vi "Start Action Core.vi"(8 "error in (no error)":errorcluster, 11 "NI DMM in":refnum<class "NI DMM.lvclass">) -> (0 "error out":errorcluster, 3 "NI DMM out":refnum<class "NI DMM.lvclass">)   [LabVIEW 2020, in "NI DMM.lvlib" / "NI DMM.lvclass"]
uses:
  NI DMM.lvclass
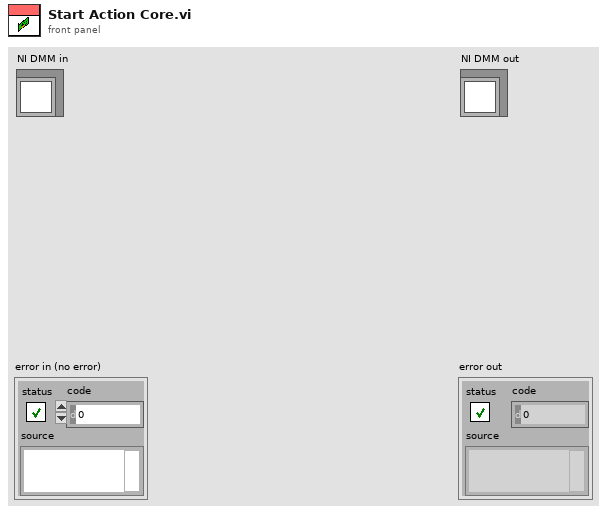
[diagram p1: front panel]
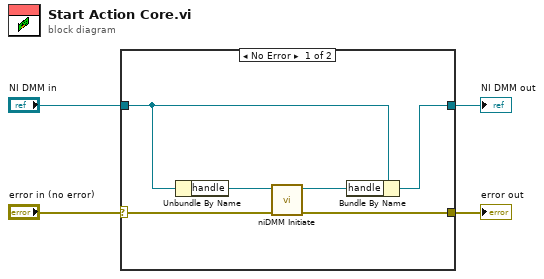
[diagram p0: block diagram]
diagram:
  n1 = case shown="No Error" "error in (no error)" {
    selector: "error in (no error)" -> [w10 w12]
    tunnel: [w6 w12] -> w3
    tunnel: "NI DMM in" -> [w8 w11]
    tunnel: [w5 w11] -> w1
    frame No Error {
      n2 = Unbundle By Name(w8) -> ("handle"=w9:refnum<k15>)
      n3 = call <instrlib>:"niDMM Initiate.vi"("error in (no error)"=w10, "instrument handle"=w9) -> ("error out"=w6:errorcluster, "instrument handle out"=w7:refnum<k15>)  [unwired: 8 in]
      n4 = Bundle By Name(cluster=w8, "handle"=w7) -> (w5:refnum<class "NI DMM.lvclass">)
    }
    frame Error {
    }
  }
  "error out" <- w3
  "NI DMM out" <- w1
